vi "Read buffer (as ByteArray).vi"(8 "error in (no error)":errorcluster, 11 "httpRequest in":refnum<class "httpRequest.lvclass">) -> (0 "error out":errorcluster, 2 "bytes":u8[](array[numeric]) format="%02x", 3 "httpRequest out":refnum<class "httpRequest.lvclass">)   [LabVIEW 2020, in "httpClient.lvlib" / "httpRequest.lvclass"]
uses:
  httpRequest.lvclass
  httpRequest.lvclass/httpRequest.ctl
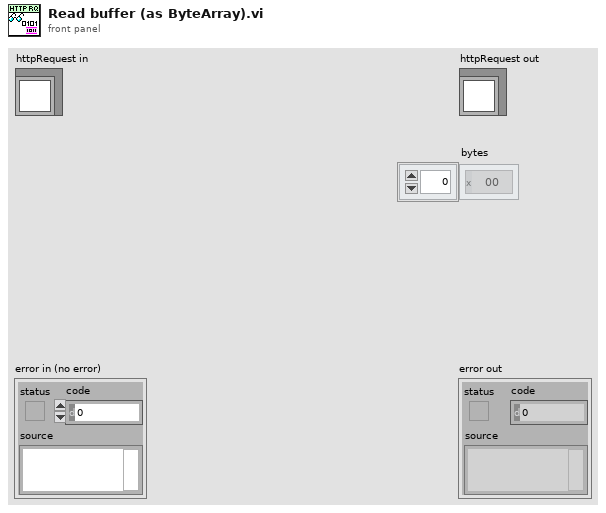
[diagram p1: front panel]
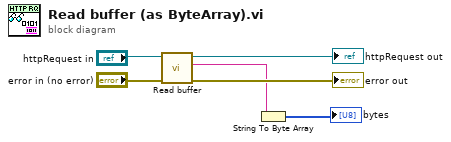
[diagram p0: block diagram]
diagram:
  n1 = call "Read buffer.vi"("error in (no error)"="error in (no error)", "httpRequest in"="httpRequest in") -> ("error out"=→"error out":errorcluster, "buffer"=w2:string, "httpRequest out"=→"httpRequest out":refnum<class "httpRequest.lvclass">)  [unwired: 7 in]
  n2 = String To Byte Array(string=w2) -> (unsigned byte array=→"bytes":u8[])
